vi "Replace DAQ Controls.vi"(0 "vi in":refnum<vi>, 11 "error in":errorcluster) -> (4 "vi out":refnum<vi>, 15 "error out":errorcluster)   [LabVIEW 2021, in "Converter.lvlib"]
uses:
  Converter.lvlib
  <vilib>/Utility/traverseref.llb/TRef TravTarget.ctl
  <vilib>/Utility/traverseref.llb/VI Scripting - Traverse.lvlib
  Path Functions/Path Functions.lvlib
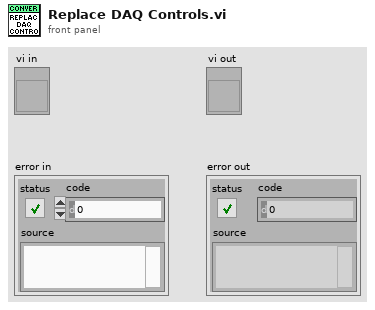
[diagram p1: front panel]
types:
  T1 = typedef "TRef TravTarget.ctl" = enum16{"FP", "BD", "Other"}
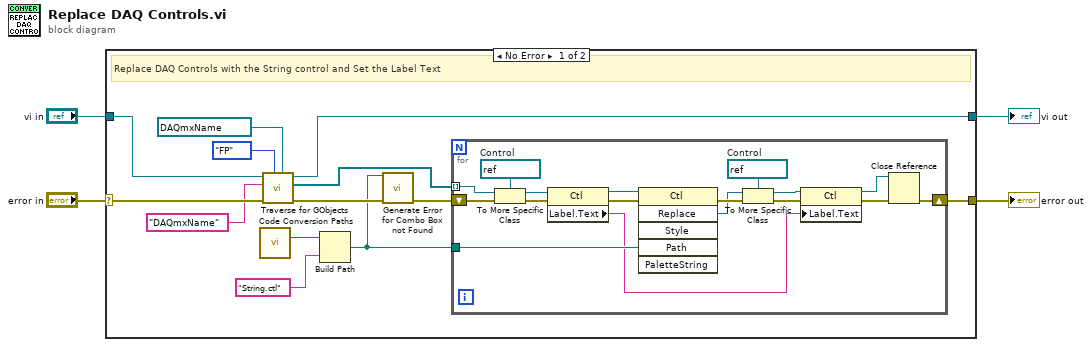
[diagram p0: block diagram]
diagram:
  n1 = case shown="No Error" "error in" {
    selector: "error in" -> [w15 w35]
    tunnel: [w8 w35] -> w4
    tunnel: [w16 w36] -> w3
    tunnel: "vi in" -> [w14 w36]
    frame No Error {
      # "Replace DAQ Controls with the String control and Set the Label Text"
      n2 = call "Code Conversion Paths.vi"() -> ("io controls"=w13:path)  [unwired: 7 in, 8 out]
      n3 = call <vilib>:"Traverse for GObjects.vi"("Other Refnum"=refnum<vi> refnum, "Traverse Target"=TRef_TravTarget."FP", "error in (no error)"=w15, "Class Name"="DAQmxName", "VI Refnum"=w14) -> ("error out"=w11:errorcluster, "References"=w9:refnum<vi>[], "dup VI Refnum"=w16:refnum<vi>)  [unwired: 3 in, 1 out]
      n4 = Build Path(base path=w13, name or relative path="String.ctl" ("string")) -> (appended path=w5:path)
      n5 = call "Generate Error for Combo Box not Found.vi"("template combox path"=w5, "error in"=w11) -> ("error out"=w10:errorcluster)  [unwired: 13 in]
      n6 = for {
        tunnel: w9 -> [w34] mode=indexing
        shift-right: [w18] -> w8
        shift-left: w10 -> [w33]
        tunnel: w5 -> [w26]
        w22 = refnum<vi> refnum  # Control
        w25 = refnum<vi> refnum  # Control
        n7 = To More Specific Class(target class=w25, reference=w34, error in=w33) -> (specific class reference=w32:refnum<vi>, error out=w30:errorcluster)
        n8 = property class="Ctl"(reference=w32, error in=w30) -> (reference out=w31:refnum<vi>, error out=w29:errorcluster, "Label.Text"=w24:string)
        n9 = invoke class="Ctl" method="Replace"(reference=w31, error in=w29, "Path"=w26) -> (error out=w28:errorcluster, "Replace"=w23:refnum<vi>)  [unwired: 3 in, 4 out]
        n10 = To More Specific Class(target class=w22, reference=w23, error in=w28) -> (specific class reference=w21:refnum<vi>, error out=w27:errorcluster)
        n11 = property class="Ctl"(reference=w21, error in=w27, "Label.Text"=w24) -> (reference out=w19:refnum<vi>, error out=w20:errorcluster)
        n12 = Close Reference(reference=w19, error in (no error)=w20) -> (error out=w18:errorcluster)
      }
    }
    frame Error {
    }
  }
  "error out" <- w4
  "vi out" <- w3
